vi "Test.vi"() -> ()   [LabVIEW 2013, in "Generic Power Supply.lvlib" / "Abstract Power Supply.lvclass"]
uses:
  Abstract Power Supply.lvclass
panel:
  in  "write buffer":string
  out "error out":errorcluster
  out "read buffer":string
  in  "VISA resource name":refnum<visa-resource-name>
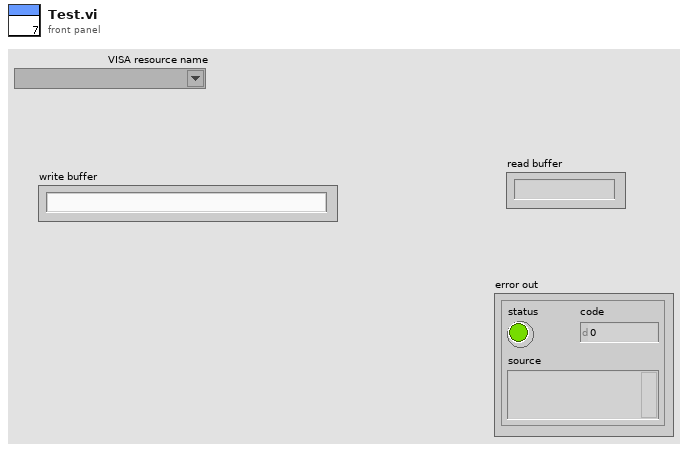
[diagram p1: front panel]
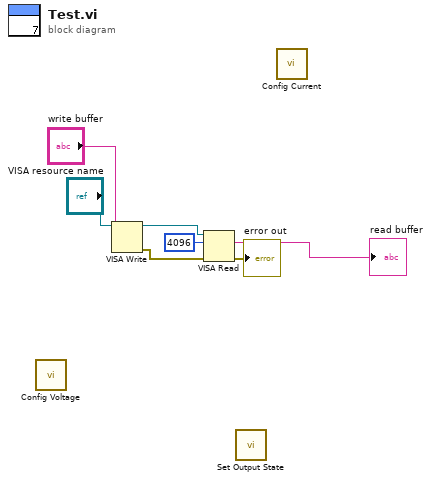
[diagram p0: block diagram]
diagram:
  n1 = call <instrlib>:"Config Voltage.vi"() -> ()  [unwired: 14 in, 2 out]
  n2 = VISA Write(VISA resource name="VISA resource name", write buffer="write buffer") -> (VISA resource name out=w6:refnum<visa-resource-name>, error out=w5:errorcluster)  [unwired: 1 in, 1 out]
  n3 = VISA Read(VISA resource name=w6, byte count=u32 4096, error in (no error)=w5) -> (read buffer=→"read buffer":string, error out=→"error out":errorcluster)  [unwired: 2 out]
  n4 = call <instrlib>:"Set Output State.vi"() -> ()  [unwired: 14 in, 2 out]
  n5 = call <instrlib>:"Config Current.vi"() -> ()  [unwired: 14 in, 2 out]
